vi "Traegergas aus Verduennungsgas.vi"(11 "Verdünnungsgas":T2 items=["N2", "O2"]) -> (3 "Trägergas":T1="N2" caption="Carrier Gas")   [LabVIEW 2020, in "Linearisierung v2.lvlib" / "SpanEinstellungen.lvlib"]
uses:
  Seiten/System Einstellungen V2/Traegergas.ctl
  SpanEinstellungen.lvlib
  Gasteiler/Gasteiler.lvlib
  Seiten/System Einstellungen V2/System Einstellungen V2.lvlib
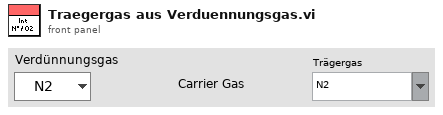
[diagram p1: front panel]
types:
  T1 = typedef "System Einstellungen V2.lvlib/Traegergas.ctl" = string
  T2 = typedef "Linearisierung v2.lvlib/Gasteiler.lvlib/Prüfgas in.ctl" = u16
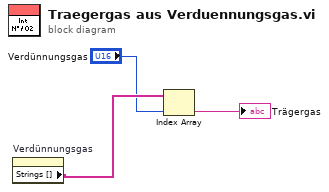
[diagram p0: block diagram]
diagram:
  n1 = property on="Verdünnungsgas" class="Ring (strikt)"() -> ("Strings []"=w3:string[])  [unwired: 2 in, 2 out]
  n2 = Index Array(array=w3, index="Verdünnungsgas") -> (element=→"Trägergas":string)
